vi "Requests.vi"(8 "error in (no error)":errorcluster, 9 "write enable":bool=TRUE, 11 "SMSD in":refnum<class "SMSD.lvclass">) -> (0 "error out":errorcluster, 3 "SMSD out":refnum<class "SMSD.lvclass">)   [LabVIEW 2021, in "SMSD.lvclass"]
uses:
  SMSD.lvclass
  SMSD.lvclass/SMSD.ctl
  Data Unit/SMSD Data Unit/ERROR_OR_COMMANT_Type.ctl
  Data Unit/SMSD Data Unit/SMSD Data Unit.lvclass
  Network Protocol/SMSD Master/SMSD Master.lvclass
  Master CR.lvclass
  Modbus_v121c/Data Model/Device Data Model.lvclass
  C:/my_projects/projects/Algorithms/Labview/21/Master CR/Master CR.lvclass
  C:/my_projects/projects/Algorithms/Labview/21/Master CR/Devices/SMSD/SMSD.lvclass
panel:
  out "position":i32
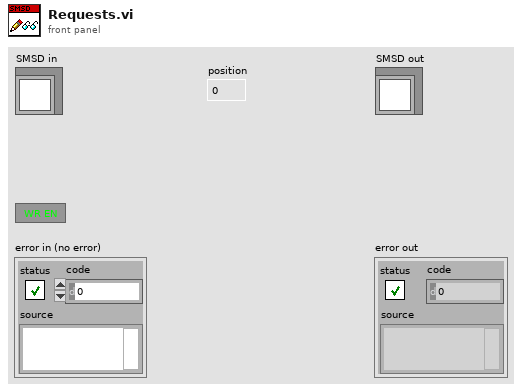
[diagram p1: front panel]
types:
  T1 = typedef "SMSD Data Unit.lvclass/ERROR_OR_COMMANT_Type.ctl" = enum8{"OK", "OK_ACCESS", "ERROR_ACCESS", "ERROR_ACCESS_TIMEOUT", "ERROR_XOR", "ERROR_NO_COMMAND", "ERROR_LEN", "ERROR_RANGE", "ERROR_WRITE", "ERROR_READ", "ERROR_PROGRAMS", "ERROR_WRITE_SETUP", "NO_NEXT", "END_PROGRAMS", "COMMAND_GET_STATUS_IN_EVENT", "COMMAND_GET_MODE", "COMMAND_GET_ABS_POS", "COMMAND_GET_EL_POS", "COMMAND_GET_SPEED", "COMMAND_GET_MIN_SPEED", "COMMAND_GET_MAX_SPEED", "COMMAND_GET_STACK", "STATUS_RELE_SET", "STATUS_RELE_CLR"}
  T2 = enum8{"CMD_PowerSTEP01_END", "CMD_PowerSTEP01_GET_SPEED", "CMD_PowerSTEP01_STATUS_IN_EVENT", "CMD_PowerSTEP01_SET_MODE", "CMD_PowerSTEP01_GET_MODE", "CMD_PowerSTEP01_SET_MIN_SPEED", "CMD_PowerSTEP01_SET_MAX_SPEED", "CMD_PowerSTEP01_SET_ACC", "CMD_PowerSTEP01_SET_DEC", "CMD_PowerSTEP01_SET_FS_SPEED", "CMD_PowerSTEP01_SET_MASK_EVENT", "CMD_PowerSTEP01_GET_ABS_POS", "CMD_PowerSTEP01_GET_EL_POS", "CMD_PowerSTEP01_GET_STATUS_AND_CLR", "CMD_PowerSTEP01_RUN_F", "CMD_PowerSTEP01_RUN_R", "CMD_PowerSTEP01_MOVE_F", "CMD_PowerSTEP01_MOVE_R", "CMD_PowerSTEP01_GO_TO_F", "CMD_PowerSTEP01_GO_TO_R", "CMD_PowerSTEP01_GO_UNTIL_F", "CMD_PowerSTEP01_GO_UNTIL_R", "CMD_PowerSTEP01_SCAN_ZERO_F", "CMD_PowerSTEP01_SCAN_ZERO_R", "CMD_PowerSTEP01_SCAN_LABEL_F", "CMD_PowerSTEP01_SCAN_LABEL_R", "CMD_PowerSTEP01_GO_ZERO", "CMD_PowerSTEP01_GO_LABEL", "CMD_PowerSTEP01_GO_TO", "CMD_PowerSTEP01_RESET_POS", "CMD_PowerSTEP01_RESET_POWERSTEP01", "CMD_PowerSTEP01_SOFT_STOP", "CMD_PowerSTEP01_HARD_STOP", "CMD_PowerSTEP01_SOFT_HI_Z", "CMD_PowerSTEP01_HARD_HI_Z", "CMD_PowerSTEP01_SET_WAIT", "CMD_PowerSTEP01_SET_RELE", "CMD_PowerSTEP01_CLR_RELE", "CMD_PowerSTEP01_GET_RELE", "CMD_PowerSTEP01_WAIT_IN0", "CMD_PowerSTEP01_WAIT_IN1", "CMD_PowerSTEP01_GOTO_PROGRAM", "CMD_PowerSTEP01_GOTO_PROGRAM_IF_IN0", "CMD_PowerSTEP01_GOTO_PROGRAM_IF_IN1", "CMD_PowerSTEP01_LOOP_PROGRAM", "CMD_PowerSTEP01_CALL_PROGRAM", "CMD_PowerSTEP01_RETURN_PROGRAM", "CMD_PowerSTEP01_START_PROGRAM_MEM0", "CMD_PowerSTEP01_START_PROGRAM_MEM1", "CMD_PowerSTEP01_START_PROGRAM_MEM2", "CMD_PowerSTEP01_START_PROGRAM_MEM3", "CMD_PowerSTEP01_STOP_PROGRAM_MEM", "CMD_PowerSTEP01_STEP_CLOCK", "CMD_PowerSTEP01_STOP_USB", "CMD_PowerSTEP01_GET_MIN_SPEED", "CMD_PowerSTEP01_GET_MAX_SPEED", "CMD_PowerSTEP01_GET_STACK", "CMD_PowerSTEP01_GOTO_PROGRAM_IF_ZERO", "CMD_PowerSTEP01_GOTO_PROGRAM_IF_IN_ZERO", "CMD_PowerSTEP01_WAIT_CONTINUE", "CMD_PowerSTEP01_SET_WAIT_2", "CMD_PowerSTEP01_SCAN_MARK2_F", "CMD_PowerSTEP01_SCAN_MARK2_R"}
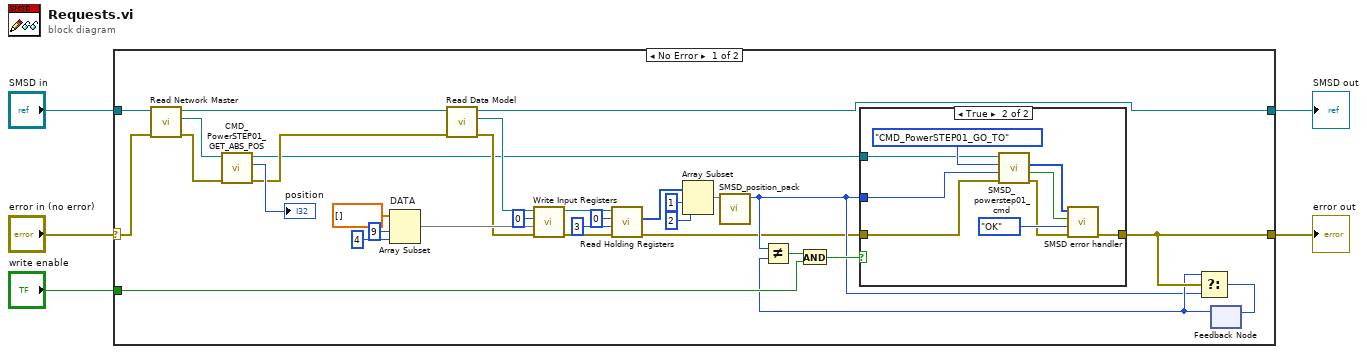
[diagram p0: block diagram]
diagram:
  n1 = case shown="No Error" "error in (no error)" {
    selector: "error in (no error)" -> [w14 w49]
    tunnel: [w32 w49] -> w1
    tunnel: [w6 w48] -> w2
    tunnel: "SMSD in" -> [w15 w48]
    tunnel: "write enable" -> [w34 _]
    frame No Error {
      n2 = call "Read Network Master.vi"("error in (no error)"=w14, "SMSD in"=w15) -> ("error out"=w12:errorcluster, "TCP Master"=w13:refnum<class "SMSD Master.lvclass">, "SMSD out"=w9:refnum<class "SMSD.lvclass">)  [unwired: 7 in]
      n3 = call "CMD_PowerSTEP01_GET_ABS_POS.vi"("error in (no error)"=w12, "SMSD in"=w13) -> ("error out"=w8:errorcluster, "position"=→"position":i32, "SMSD out"=w7:refnum<class "SMSD Master.lvclass">)  [unwired: 7 in]
      n4 = Array Subset "DATA"(array=dbl[] [], index=9, length=4) -> (w24:dbl[])
      n5 = call "Read Data Model.vi"("error in (no error)"=w8, "Master CR in"=w9) -> ("error out"=w22:errorcluster, "Data Model"=w25:refnum<class "Device Data Model.lvclass">, "Master CR out"=w6:refnum<class "SMSD.lvclass">)  [unwired: 7 in]
      n6 = call-dynamic "Write Input Registers.vi"("error in (no error)"=w22, "register values"=w24, "starting address"=u16 0, "Device Data Model in"=w25) -> ("error out"=w21:errorcluster, "Device Data Model out"=w18:refnum<class "Device Data Model.lvclass">)  [unwired: 6 in]
      n7 = call-dynamic "Read Holding Registers.vi"("error in"=w21, "number of registers"=u16 3, "starting address"=u16 0, "device data model in"=w18) -> ("error out"=w20:errorcluster, "data"=w19:u16[])  [unwired: 5 in, 1 out]
      n8 = Array Subset(array=w19, index=1, length=2) -> (w26:u16[])
      n9 = call "SMSD_position_pack.vi"("DATA"=w26) -> ("position"=w29:u32)  [unwired: 10 in]
      n10 = feedback #1() -> (w31:u32)  [unwired: 1 in]
      n11 = Not Equal?(x=w29, y=w31) -> (x != y?=w35:bool)
      n12 = And(x=w35, y=w34) -> (x .and. y?=w33:bool)
      n13 = case shown="True" w33 {
        tunnel: [w38 w43] -> w32
        tunnel: w20 -> [w38 w42]
        tunnel: w29 -> [_ w40]
        tunnel: w7 -> [_ w39]
        frame False {
        }
        frame True {
          n14 = call "SMSD_powerstep01_cmd.vi"("error in (no error)"=w42, "DATA (0)"=w40, "COMMAND (END)"=T2."CMD_PowerSTEP01_GO_TO", "SMSD in"=w39) -> ("error out"=w44:errorcluster, "PDU valid?"=w45:bool, "data"=w47:u8[])  [unwired: 4 in, 1 out]
          n15 = call "SMSD error handler.vi"("error in (no error)"=w44, "correct answer (OK)"=ERROR_OR_COMMANT_Type."OK" ("coerced x 2"), "timed out?"=w45, "data"=w47) -> ("error out"=w43:errorcluster)  [unwired: 7 in]
        }
      }
      n16 = Select(t=w31, s=w32, f=w29) -> (s? t:f=w30:u32)
      n17 = feedback-in #1(w30) -> ()
    }
    frame Error {
    }
  }
  "error out" <- w1
  "SMSD out" <- w2
